vi "OAT DC Gap Estimator.vi"   [LabVIEW 2017, in "SoundVib_RefDataProcess.lvlib"]
doc: "Subtracts the gap reference from the averaged DC gap voltage of the <B>even-angle signal</B> and returns the DC gap in the selected units. The DC gap is a measurement of the movement of the shaft from the reference position to the current position. If <B>gap reference [V]</B> is unwired, the VI computes the <B>actual gap ref [V]</B> from the input signal. Wire data to the <B>even-angle signal</B> input to determine the polymorphic instance to use or manually select the instance."
uses:
  <vilib>/addons/Sound and Vibration/Order Analysis/Referece Data Processing/SoundVib_RefDataProcess.lvlib
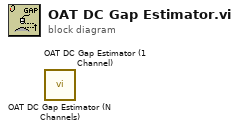
[diagram p0: block diagram]
diagram:
  n1 = call <vilib>:"OAT DC Gap Estimator (N Channels).vi"() -> ()  [unwired: 15 in, 5 out]
  n2 = call <vilib>:"OAT DC Gap Estimator (1 Channel).vi"() -> ()  [unwired: 15 in, 5 out]
